vi "Print.vi"(9 "Boolean":bool, 10 "String":string, 11 "OfficeTron3000 In":refnum<class "OfficeTron3000.lvclass">) -> (3 "OfficeTron3000 Out":refnum<class "OfficeTron3000.lvclass">)   [LabVIEW 2018, in "OfficeTron3000.lvlib" / "OfficeTron3000.lvclass"]
uses:
  OfficeTron3000.lvclass
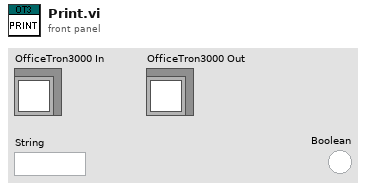
[diagram p1: front panel]
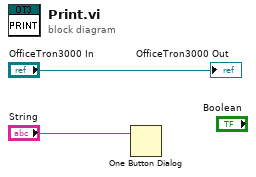
[diagram p0: block diagram]
diagram:
  n1 = One Button Dialog(message="String") -> ()  [unwired: 1 in, 1 out]
  "OfficeTron3000 Out" <- "OfficeTron3000 In"
